vi "PrepareHWI.vi"(8 "error in (no error)":errorcluster, 9 "Master Device in":refnum<class "Master Device.lvclass">, 10 "Current Variables":T1[](array[typedef]), 11 "Novatech in":refnum<class "Novatech.lvclass">) -> (0 "error out":errorcluster, 2 "Master Device out":refnum<class "Master Device.lvclass">, 3 "Novatech out":refnum<class "Novatech.lvclass">)   [LabVIEW 2013, in "Novatech.lvclass"]
uses:
  Novatech.lvclass
  TypeDefs/Active procedure variables.ctl
  Master Device/Master Device.lvclass
  Novatech.lvclass/Novatech.ctl
  Novatech 409A.lvlib
panel:
  # "This VI handles the initial creation of ramps and pruning the data (takes over the function of the PruneRamp VI which just   __identified__ the trigger lines that required updates)"
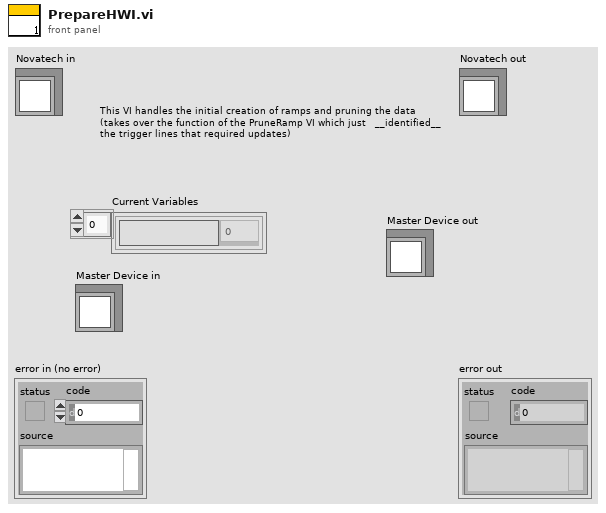
[diagram p1: front panel]
types:
  T1 = typedef "Active procedure variables.ctl" = cluster{"Procedure variable":string, "Value":dbl}
  T2 = cluster{"Triggering":bool[][], "Ramp Info":cluster{"Ramp Index":i32, "Ramp Time":dbl, "Number of Steps":i32}[], "VLIW Array":cluster{"Output Bits":u32, "Data Field":u32, "OP Code":u8, "Delay Count":u64}[]}
  T3 = cluster{"Ramp Index":i32, "Ramp Time":dbl, "Number of Steps":i32}[]
  T4 = cluster{"Nova Update List":dbl[][], "2 Freq. [MHz]":dbl, "2 Power [dBm]":u16, "2 phase":u16, "3 Freq. [MHz]":dbl, "3 Power [dBm]":u16, "3 phase":u16}[]
  T5 = cluster{"Nova Update List":dbl[][], "2 Freq. [MHz]":dbl, "2 Power [dBm]":u16, "2 phase":u16, "3 Freq. [MHz]":dbl, "3 Power [dBm]":u16, "3 phase":u16}
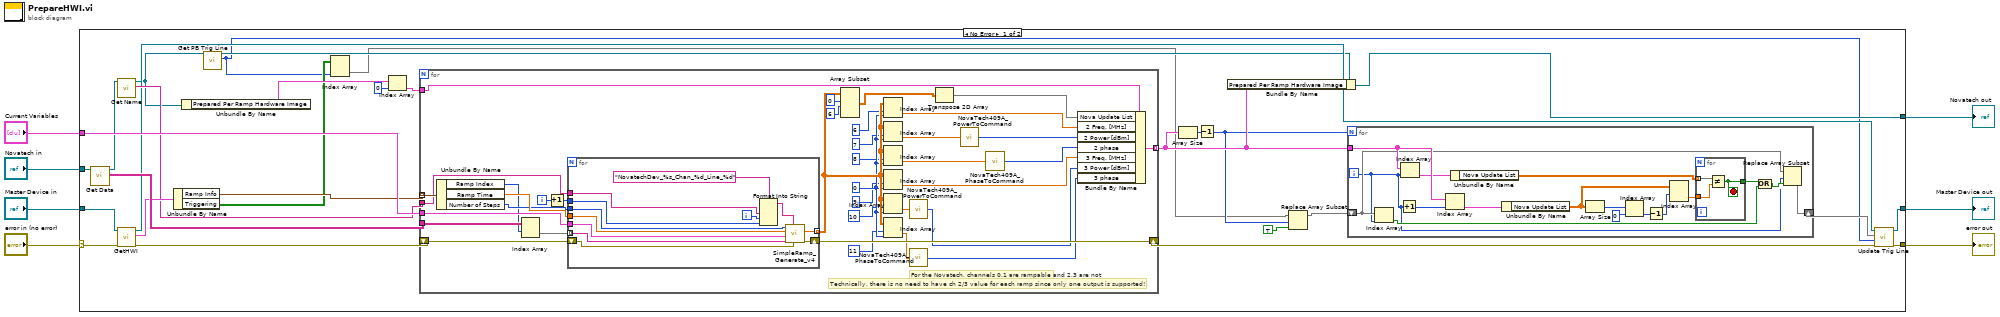
[diagram p0: block diagram]
diagram:
  n1 = case shown="No Error" "error in (no error)" {
    selector: "error in (no error)" -> [w32 w107]
    tunnel: "Current Variables" -> [w34 _]
    tunnel: [w13 w106] -> w4
    tunnel: [w25 w107] -> w6
    tunnel: "Novatech in" -> [w36 w106]
    tunnel: "Master Device in" -> [w33 w105]
    tunnel: [w26 w105] -> w1
    frame No Error {
      n2 = call-dynamic "Get Data.vi"("Device in"=w36) -> ("Table Indicator"=w35:string[][], "Device out"=w29:refnum<class "Novatech.lvclass">)  [unwired: 7 in, 1 out]
      n3 = call-dynamic "Get Name.vi"("Device in"=w29) -> ("Name"=w28:string, "Device out"=w15:refnum<class "Novatech.lvclass">)  [unwired: 8 in, 1 out]
      n4 = call-dynamic "GetHWI.vi"("error in (no error)"=w32, "Master Device in"=w33) -> ("error out"=w31:errorcluster, "Hardware Image"=w30:T2, "Master Device out"=w27:refnum<class "Master Device.lvclass">)  [unwired: 7 in]
      n5 = Unbundle By Name(w30) -> ("Ramp Info"=w21:T3, "Triggering"=w11:bool[][])
      n6 = Unbundle By Name(w15) -> ("Prepared Per Ramp Hardware Image"=w19:T4)
      n7 = call-dynamic "Get PB Trig Line.vi"("Device in"=w15) -> ("PB Trigger Line"=w8:u16, "Device out"=w14:refnum<class "Novatech.lvclass">)  [unwired: 8 in, 1 out]
      n8 = Index Array(array=w11, index (col)=w8) -> (element=w10:bool[])  [unwired: 1 in]
      n9 = Index Array(array=w19, index=0) -> (element=w20:T5)
      n10 = for {
        tunnel: w35 -> [w61]
        tunnel: w34 -> [w91]
        shift-right: [w92] -> w12
        shift-left: w31 -> [w90]
        tunnel: w21 -> [w67] mode=indexing
        tunnel: [w64] -> w23 mode=indexing
        tunnel: w28 -> [w63]
        tunnel: w20 -> [w59]
        i -> [w58]
        w82 = 0
        # "Technically, there is no need to have ch 2/3 value for each ramp since only one output is supported!"
        # "For the Novatech, channels 0,1 are rampable and 2,3 are not"
        n11 = Unbundle By Name(w67) -> ("Ramp Index"=w60:i32, "Ramp Time"=w66:dbl, "Number of Steps"=w65:i32)
        n12 = Index Array(array=w61, index (row)=w60) -> (element=w62:string[])  [unwired: 1 in]
        n13 = Increment(x=w58) -> (x+1=w57:i32)
        n14 = for {
          tunnel: [w104] -> w85 mode=indexing
          tunnel: w62 -> [w94] mode=indexing
          shift-right: [w103] -> w92
          shift-left: w90 -> [w102]
          tunnel: w91 -> [w101]
          tunnel: w66 -> [w100]
          tunnel: w65 -> [w99]
          tunnel: w63 -> [w97]
          tunnel: w57 -> [w95]
          i -> [w96]
          n15 = Format Into String(format string="NovatechDev_%s_Chan_%d_Line_%d", w97, w96, w95) -> (resulting string=w93:string)  [unwired: 2 in, 1 out]
          n16 = call "SimpleRamp_Generate_v4.vi"("error in (no error)"=w102, "Error Locator"=w93, "formula"=w94, "Current Variable settings"=w101, "dt"=w100, "Points"=w99) -> ("error out"=w103:errorcluster, "y values"=w104:dbl[])  [unwired: 1 in, 1 out]
        }
        n17 = Array Subset(array=w85, index (row)=0 ("index"), length (row)=6 ("length")) -> (w88:dbl[][])  [unwired: 2 in]
        n18 = Index Array(array=w85, index (row)=6, index (col)=w82) -> (element=w87:dbl)
        n19 = Index Array(array=w85, index (row)=7, index (col)=w82) -> (element=w75:dbl)
        n20 = Index Array(array=w85, index (row)=8, index (col)=w82) -> (element=w73:dbl)
        n21 = Index Array(array=w85, index (row)=9, index (col)=w82) -> (element=w86:dbl)
        n22 = Index Array(array=w85, index (row)=10, index (col)=w82) -> (element=w71:dbl)
        n23 = Index Array(array=w85, index (row)=11, index (col)=w82) -> (element=w69:dbl)
        n24 = call "NovaTech409A_PowerToCommand.vi"("Novatech Power [dBm]"=w71) -> ("Novatech Command"=w70:u16)
        n25 = call "NovaTech409A_PhaseToCommand.vi"("Novatech Phase [Degrees]"=w69) -> ("Novatech Command"=w68:u16)
        n26 = Transpose 2D Array(2D array=w88) -> (transposed array=w89:dbl[][])
        n27 = call "NovaTech409A_PowerToCommand.vi"("Novatech Power [dBm]"=w75) -> ("Novatech Command"=w74:u16)
        n28 = call "NovaTech409A_PhaseToCommand.vi"("Novatech Phase [Degrees]"=w73) -> ("Novatech Command"=w72:u16)
        n29 = Bundle By Name(cluster=w59, "Nova Update List"=w89, "2 Freq. [MHz]"=w87, "2 Power [dBm]"=w74, "2 phase"=w72, "3 Freq. [MHz]"=w86, "3 Power [dBm]"=w70, "3 phase"=w68) -> (w64:T5)
      }
      n30 = Array Size(array=w23) -> (size(s)=w24:i32)
      n31 = Decrement(x=w24) -> (x-1=w16:i32)
      n32 = Bundle By Name(cluster=w14, "Prepared Per Ramp Hardware Image"=w23) -> (w13:refnum<class "Novatech.lvclass">)
      n33 = Replace Array Subset(array=w10, new element=TRUE ("new element/subarray"), index=w16) -> (w17:bool[])
      n34 = for {
        N: w16 -> [_]
        tunnel: w23 -> [w44]
        shift-right: [w41] -> w22
        shift-left: w17 -> [w42]
        i -> [w37]
        n35 = Index Array(array=w42, index=w37) -> (element=w48:bool)
        n36 = Increment(x=w37) -> (x+1=w38:i32)
        n37 = Index Array(array=w44, index=w37) -> (element=w43:T5)
        n38 = Index Array(array=w44, index=w38) -> (element=w45:T5)
        n39 = Unbundle By Name(w43) -> ("Nova Update List"=w50:dbl[][])
        n40 = Unbundle By Name(w45) -> ("Nova Update List"=w51:dbl[][])
        n41 = Array Size(array=w51) -> (size(s)=w53:i32[])
        n42 = Index Array(array=w53, index=0) -> (element=w47:i32)
        n43 = Decrement(x=w47) -> (x-1=w46:i32)
        n44 = Index Array(array=w51, index (row)=w46) -> (element=w49:dbl[])  [unwired: 1 in]
        n45 = for {
          tunnel: w50 -> [w55] mode=indexing
          tunnel: w49 -> [w56]
          tunnel: [w54] -> w39
          stop <- w54 stop-if-true
          n46 = Not Equal?(x=w55, y=w56) -> (x != y?=w54:bool)
        }
        n47 = Or(x=w39, y=w48) -> (x .or. y?=w40:bool)
        n48 = Replace Array Subset(array=w42, new element=w40, index=w37) -> (w41:bool[])
      }
      n49 = call-dynamic "Update Trig Line.vi"("error in (no error)"=w12, "PB Trigger Line"=w8, "Triggering"=w22, "Master Device in"=w27) -> ("error out"=w25:errorcluster, "Master Device out"=w26:refnum<class "Master Device.lvclass">)  [unwired: 6 in]
    }
    frame Error {
    }
  }
  "error out" <- w6
  "Novatech out" <- w4
  "Master Device out" <- w1
